vi "FULLADDER.vi"() -> ()   [LabVIEW 2018]
panel:
  out "carry":bool
  out "sum":bool
  in  "?":bool
  in  "?":bool
  in  "?":bool
  # "full adder"
  # "a"
  # "b"
  # "c"
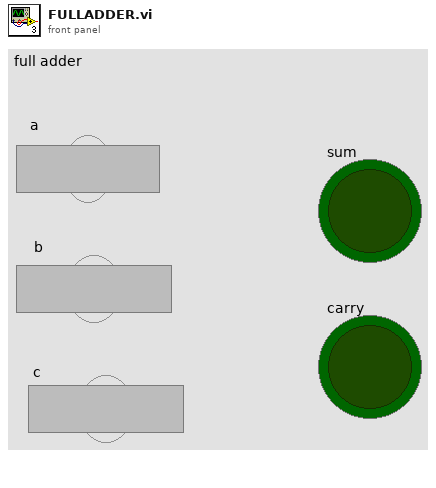
[diagram p1: front panel]
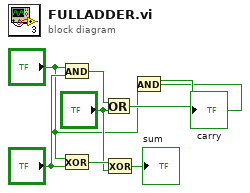
[diagram p0: block diagram]
diagram:
  n1 = And(x="?", y="?") -> (x .and. y?=w5:bool)
  n2 = Exclusive Or(1:"?", 2:"?") -> (0:w8:bool)
  n3 = Or(x=w5, y="?") -> (x .or. y?=w3:bool)
  n4 = Exclusive Or(1:"?", 2:w8) -> (0:→"sum":bool)
  n5 = And(x=w3, y="?") -> (x .and. y?=→"carry":bool)
